vi "Goal Mode Filter 624 Aerial Assist.vi"(5 "Left Cam?":bool, 9 "Targets In":T2(array[cluster]), 10 "Vision Mode":T3) -> (2 "Targets Out":T2(array[cluster]))   [LabVIEW 2013]
uses:
  Common Code/Vision Mode.ctl
  TargetType.ctl
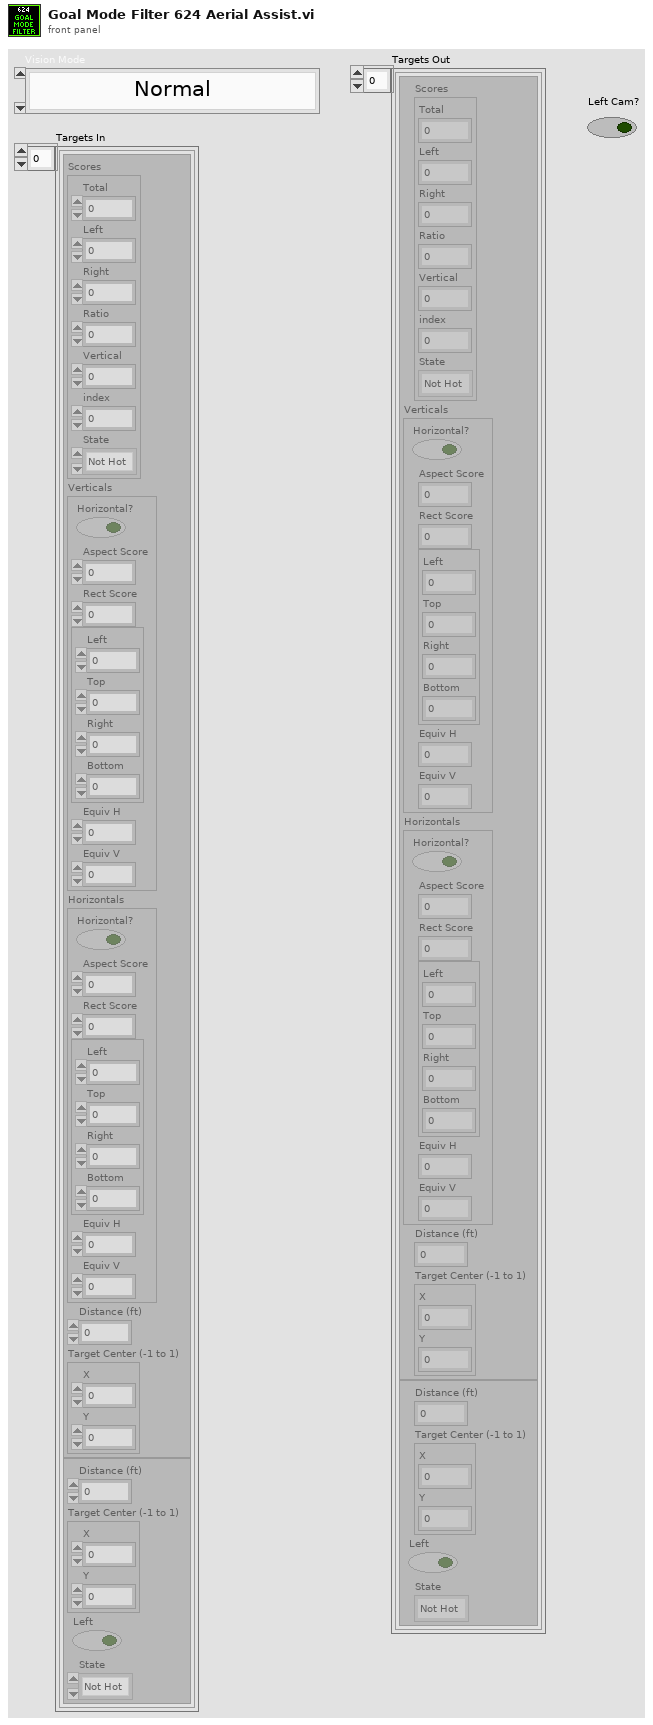
[diagram p1: front panel]
types:
  T1 = typedef "TargetType.ctl" = enum16{"Not Hot", "Hot"}
  T2 = cluster{cluster{"Scores":cluster{"Total":dbl, "Left":dbl, "Right":dbl, "Ratio":dbl, "Vertical":dbl, "index":i32, "State":T1}, "Verticals":cluster{"Horizontal?":bool, "Aspect Score":dbl, "Rect Score":dbl, cluster{"Left":dbl, "Top":dbl, "Right":dbl, "Bottom":dbl}, "Equiv H":dbl, "Equiv V":dbl}, "Horizontals":cluster{"Horizontal?":bool, "Aspect Score":dbl, "Rect Score":dbl, cluster{"Left":dbl, "Top":dbl, "Right":dbl, "Bottom":dbl}, "Equiv H":dbl, "Equiv V":dbl}, "Distance (ft)":dbl, "Target Center (-1 to 1)":cluster{"X":dbl, "Y":dbl}}, cluster{"Distance (ft)":dbl, "Target Center (-1 to 1)":cluster{"X":dbl, "Y":dbl}, "Left":bool, "State":T1}}[]
  T3 = typedef "Vision Mode.ctl" = enum16{"Normal", "Extreme Left", "Extreme Right"}
  T4 = cluster{cluster{"Distance (ft)":dbl, "Target Center (-1 to 1)":cluster{"X":dbl, "Y":dbl}, "Left":bool, "State":T1}}
  T5 = cluster{"Distance (ft)":dbl, "Target Center (-1 to 1)":cluster{"X":dbl, "Y":dbl}, "Left":bool, "State":T1}
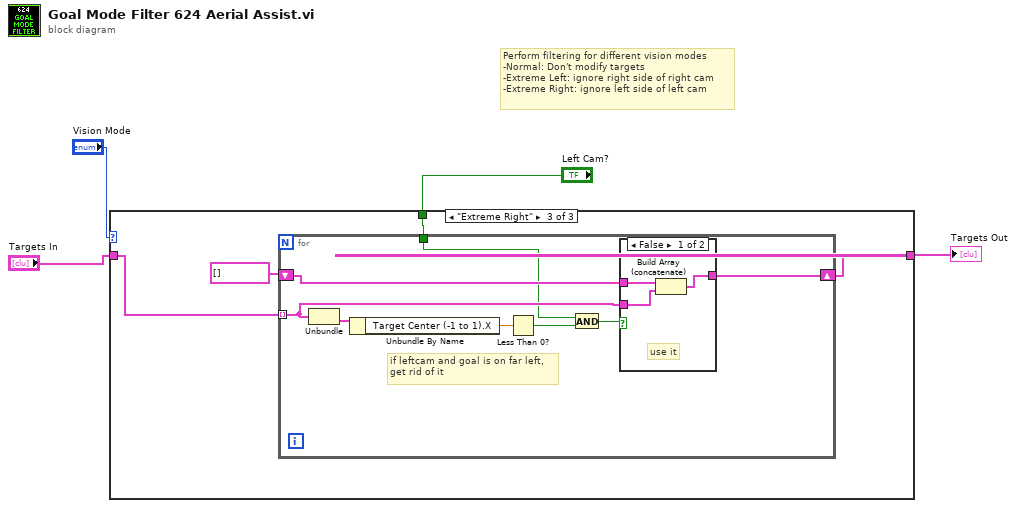
[diagram p0: block diagram]
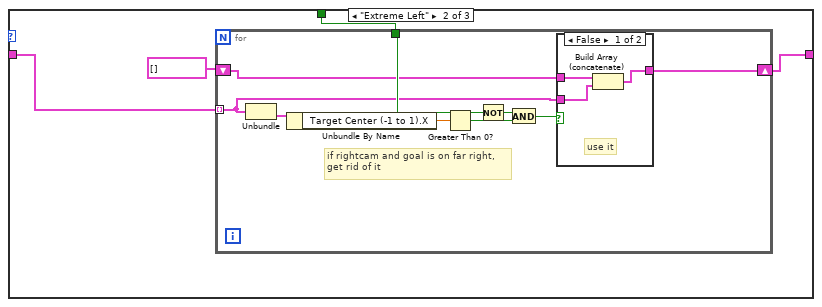
[diagram p3: hidden frame]
diagram:
  # "Perform filtering for different vision modes\n-Normal: Don't modify targets\n-Extreme Left: ignore right side of right cam\n-Extreme Right: ignore left side of left cam"
  n1 = case shown="\"Extreme Right\"" "Vision Mode" {
    tunnel: "Targets In" -> [w5 w9 w25]
    tunnel: [w5 w6 w24] -> w3
    tunnel: "Left Cam?" -> [_ w8 w23]
    frame "Normal", Default {
      # "Leave goals alone"
    }
    frame "Extreme Left" {
      (unwired) T4 {{"Distance (ft)"=0.0, "Target Center (-1 to 1)"={"X"=0.0, "Y"=0.0}, "Left"=FALSE, "State"=enum."Not Hot"}}
      n2 = for {
        tunnel: w9 -> [w12] mode=indexing
        tunnel: w8 -> [w14]
        shift-right: [w11] -> w6
        shift-left: T2 [] -> [w10]
        # "if rightcam and goal is on far right,\nget rid of it"
        n3 = Unbundle(w12) -> (w18:T5)  [unwired: 1 out]
        n4 = Unbundle By Name(w18) -> ("Target Center (-1 to 1).X"=w17:dbl)
        n5 = Greater Than 0?(x=w17) -> (x > 0?=w16:bool)
        n6 = Not(x=w14) -> (.not. x?=w15:bool)
        n7 = And(x=w15, y=w16) -> (x .and. y?=w13:bool)
        n8 = case shown="False" w13 {
          tunnel: w12 -> [w21 _]
          tunnel: [w20 w22] -> w11
          tunnel: w10 -> [w19 w22]
          frame False {
            # "use it"
            n9 = Build Array (concatenate)(w19, w21) -> (w20:T2)
          }
          frame True {
            # "don't use it"
          }
        }
      }
    }
    frame "Extreme Right" {
      n10 = for {
        tunnel: w25 -> [w30] mode=indexing
        shift-right: [w29] -> w24
        shift-left: T2 [] -> [w28]
        tunnel: w23 -> [w27]
        # "if leftcam and goal is on far left,\nget rid of it"
        n11 = Unbundle(w30) -> (w34:T5)  [unwired: 1 out]
        n12 = Unbundle By Name(w34) -> ("Target Center (-1 to 1).X"=w33:dbl)
        n13 = Less Than 0?(x=w33) -> (x < 0?=w32:bool)
        n14 = And(x=w27, y=w32) -> (x .and. y?=w31:bool)
        n15 = case shown="False" w31 {
          tunnel: w30 -> [w37 _]
          tunnel: [w36 w38] -> w29
          tunnel: w28 -> [w35 w38]
          frame False {
            # "use it"
            n16 = Build Array (concatenate)(w35, w37) -> (w36:T2)
          }
          frame True {
            # "don't use it"
          }
        }
      }
    }
  }
  "Targets Out" <- w3
